vi "Part 2.vi"(11 "Input":string) -> (3 "Output":i64)   [LabVIEW 2021]
uses:
  <userlib>/_OpenG.lib/string/string.llb/Convert EOLs (String)__ogtk.vi
  <vilib>/regexp/Match Regular Expression.xnode
panel:
  out "Array":i64[](array[numeric])
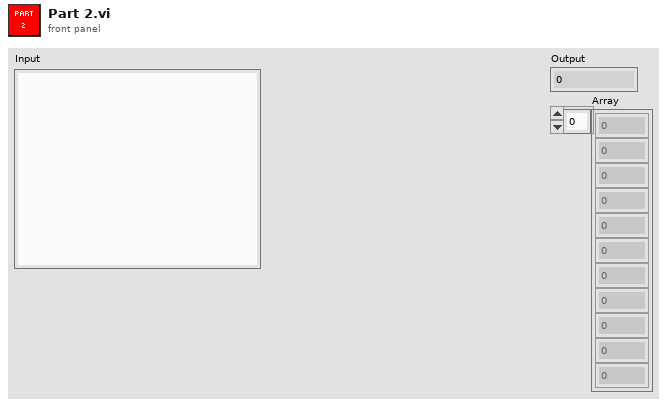
[diagram p1: front panel]
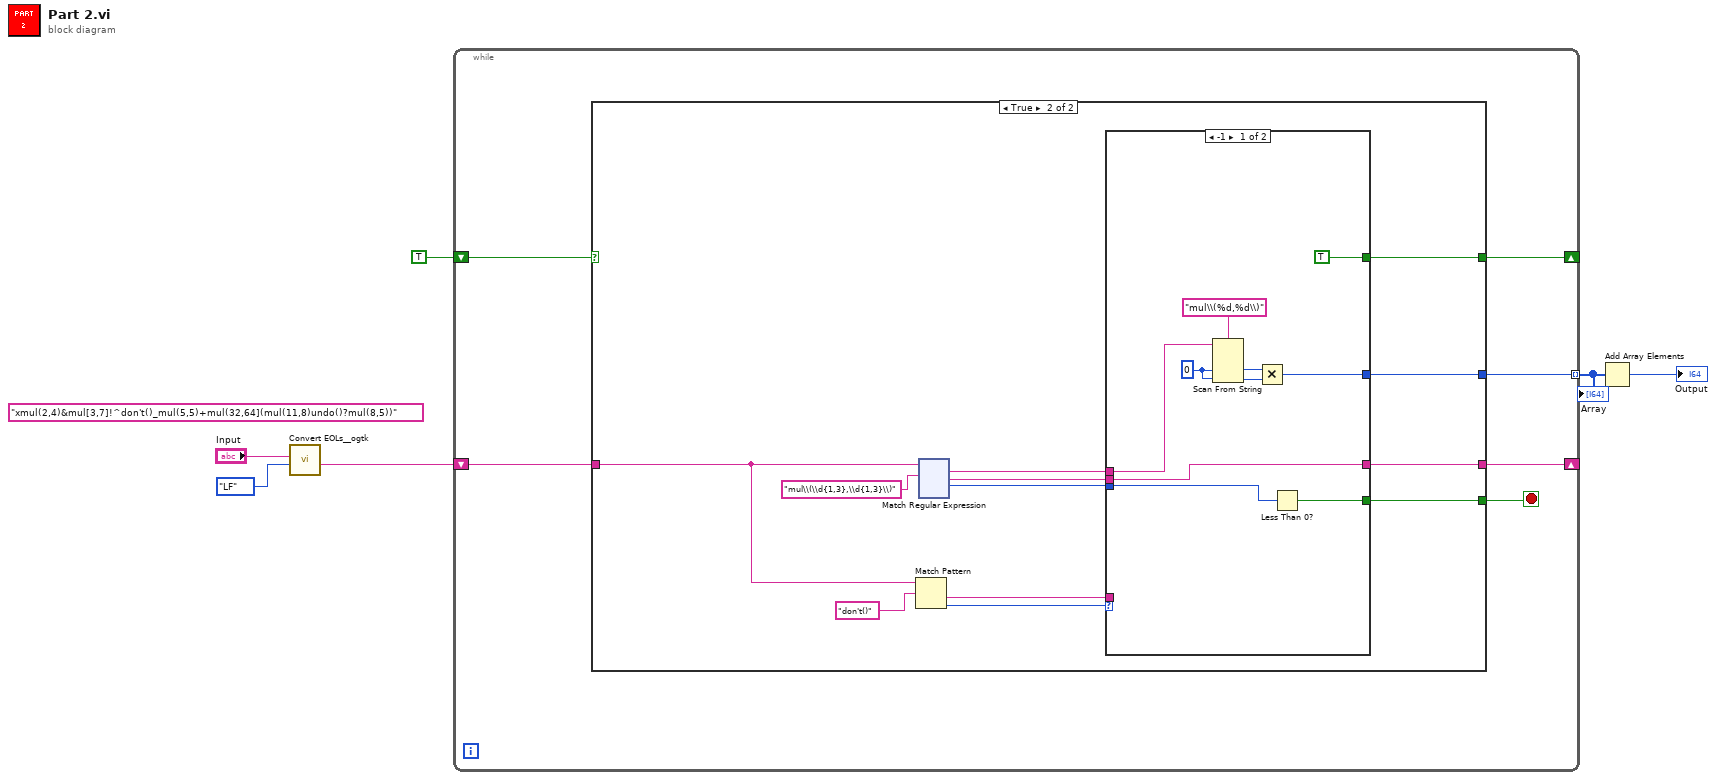
[diagram p0: block diagram]
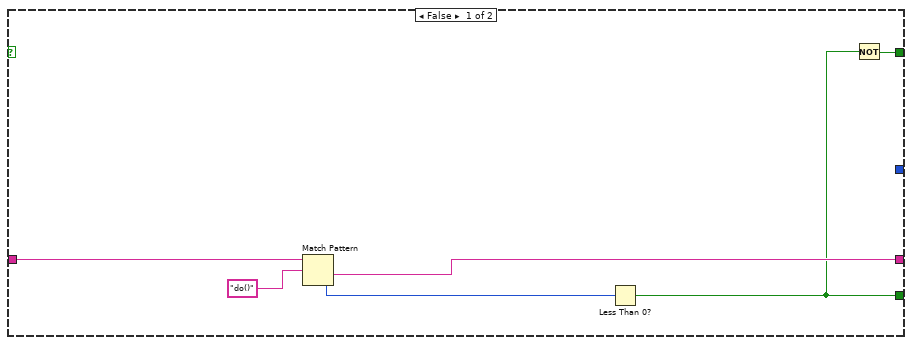
[diagram p2: hidden frame]
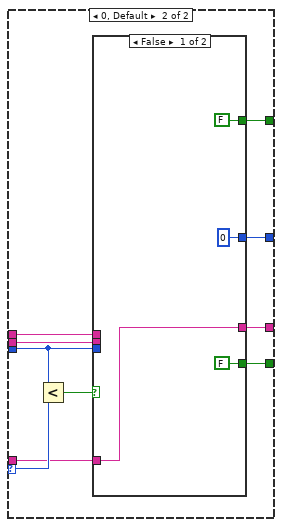
[diagram p3: hidden frame]
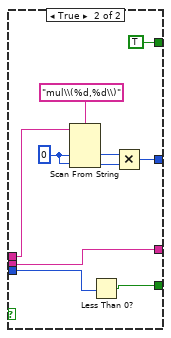
[diagram p4: hidden frame]
diagram:
  (unwired) "xmul(2,4)&mul[3,7]!^don't()_mul(5,5)+mul(32,64](mul(11,8)undo()?mul(8,5))"
  n1 = call-poly <userlib>:"Convert EOLs__ogtk.vi"("Convert to:"=enum16{"CR", "LF", "CRLF"}."LF", "String in"="Input") -> ("String out"=w5:string)  [unwired: 9 in]
  n2 = while {
    shift-right: [w11] -> _
    shift-left: w5 -> [w12]
    tunnel: [w10] -> w4 mode=indexing
    shift-right: [w7] -> _
    shift-left: TRUE -> [w9]
    stop <- w8 stop-if-true
    n3 = case shown="True" w9 {
      tunnel: w12 -> [w18 w27]
      tunnel: [w16 w22] -> w11
      tunnel: [_ w28] -> w10
      tunnel: [w13 w21] -> w8
      tunnel: [w14 w20] -> w7
      frame False {
        n4 = Match Pattern(string=w18, regular expression="do()") -> (after substring=w16:string, offset past match=w15:i32)  [unwired: 1 in, 2 out]
        n5 = Less Than 0?(x=w15) -> (x < 0?=w13:bool)
        n6 = Not(x=w13) -> (.not. x?=w14:bool)
      }
      frame True {
        n7 = Match Pattern(string=w27, regular expression="don't()") -> (after substring=w19:string, offset past match=w25:i32)  [unwired: 1 in, 2 out]
        n8 = xnode "Match Regular Expression"("input string"=w27, "regular expression"="mul\\(\\d{1,3},\\d{1,3}\\)") -> ("whole match"=w29:string, "after match"=w23:string, "offset past match"=w24:i32)  [unwired: 4 in, 2 out]
        n9 = case shown="-1" w25 {
          selector: w25 -> [_ w48]
          tunnel: w29 -> [w36 w50]
          tunnel: [w35 w49] -> w28
          tunnel: w24 -> [w33 w44]
          tunnel: w23 -> [w34 w46]
          tunnel: [w34 w45] -> w22
          tunnel: [w32 w43] -> w21
          tunnel: [TRUE w42] -> w20
          tunnel: w19 -> [_ w41]
          frame -1 {
            w37 = i64 0
            n10 = Scan From String(format string="mul\\(%d,%d\\)", input string=w36, default 1=w37, default 2=w37) -> (output 1=w38:i64, output 2=w39:i64)  [unwired: 2 in, 3 out]
            n11 = Multiply(x=w38, y=w39) -> (x*y=w35:i64)
            n12 = Less Than 0?(x=w33) -> (x < 0?=w32:bool)
          }
          frame 0, Default {
            n13 = Less?(x=w44, y=w48) -> (x < y?=w47:bool)
            n14 = case shown="False" w47 {
              tunnel: w50 -> [_ w64]
              tunnel: [i64 0 w60] -> w49
              tunnel: w46 -> [_ w58]
              tunnel: [w52 w58] -> w45
              tunnel: w44 -> [_ w57]
              tunnel: [FALSE w56] -> w43
              tunnel: [FALSE TRUE] -> w42
              tunnel: w41 -> [w52 _]
              frame False {
              }
              frame True {
                w59 = i64 0
                n15 = Scan From String(format string="mul\\(%d,%d\\)", input string=w64, default 1=w59, default 2=w59) -> (output 1=w61:i64, output 2=w62:i64)  [unwired: 2 in, 3 out]
                n16 = Less Than 0?(x=w57) -> (x < 0?=w56:bool)
                n17 = Multiply(x=w61, y=w62) -> (x*y=w60:i64)
              }
            }
          }
        }
      }
    }
  }
  "Array" <- w4
  n18 = Add Array Elements(numeric array=w4) -> (sum=→"Output":i64)
